vi "main.vi"() -> ()   [LabVIEW 2023]
uses:
  <vilib>/vision/Image Controls.llb/IMAQ Image.ctl
  <vilib>/vision/NI_Vision_Development_Module.lvlib
  <vilib>/vision/Pattern Matching.llb/IMAQ Match Range Setting.ctl
  <vilib>/vision/Shape Detection.llb/ShapeDetectionMatchOptions.ctl
  <vilib>/addons/database/NI_Database_API.lvlib
  <vilib>/addons/database/Command.llb/Cmd Set Parameter Value (C).vi
  <vilib>/addons/database/Connection.llb/DB Tools Open Connec (String).vi
  <vilib>/addons/database/Command.llb/Cmd Execute.vi
  <vilib>/addons/database/Recordset.llb/Rec Destroy - Command.vi
  <vilib>/addons/database/Command.llb/Cmd Delete.vi
panel:
  in  "Parameterized SQL query":string="insert into inserttable (querytype, device, numsamples) values ('parameterized sql query', ?, ?) "
  in  "Analiza Pythongowa":bool
  out "Shape Report":T1(array[cluster]) {"Score" format="%.2f"; "Centroid"."y" format="%.2f"; "Centroid"."x" format="%.2f"}
  out "Triangles":i32
  out "String":string
  out "Rectangles":i32
  out "Circles":i32
  out "Obraz":T2(plugin-control)
  in  "Output Path":path
  in  "Input Path":path=path "C:/Users/kacpe/Desktop/OSP/testp.png"
  in  "Refresh Button":bool
  in  "Process Stop Button":bool
  in  "Save As Button":bool
  in  "Analiza Labview":bool
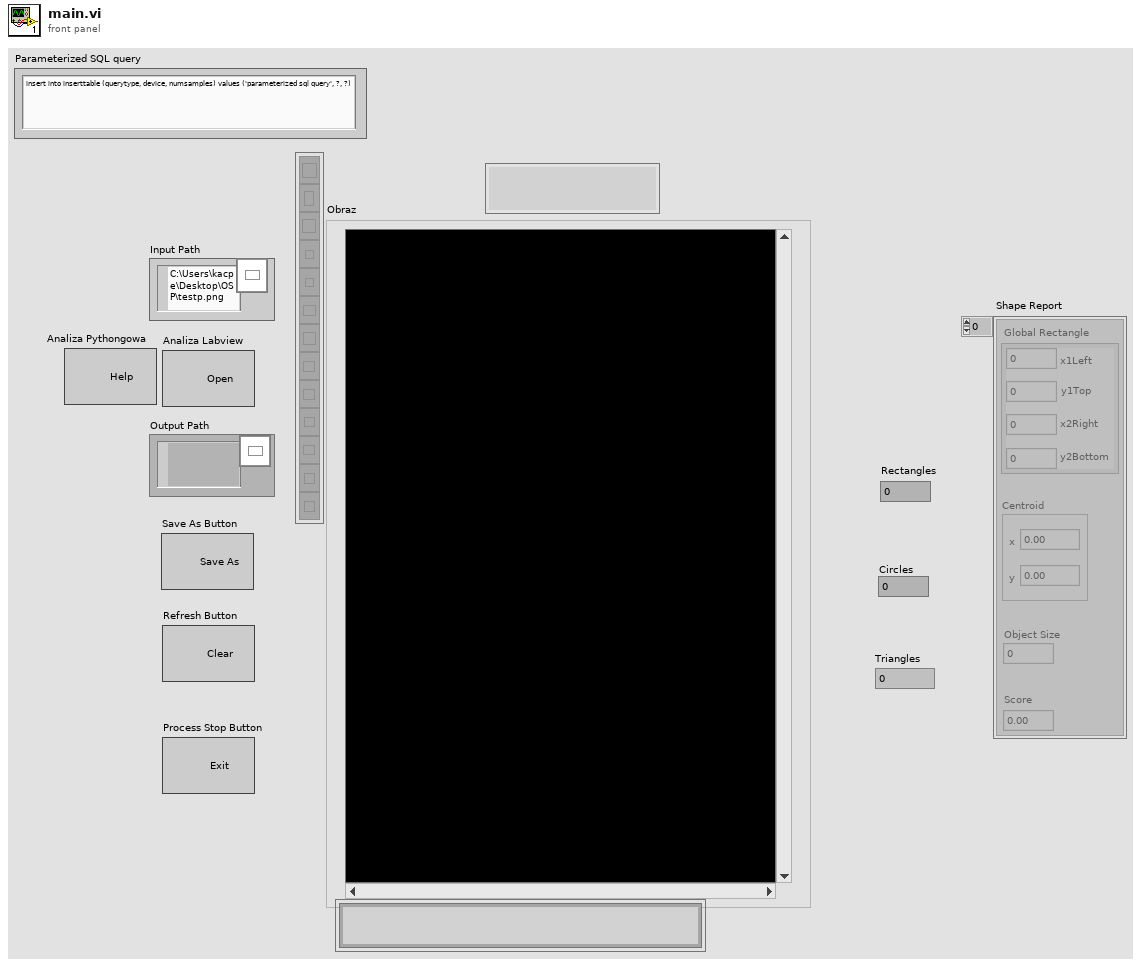
[diagram p1: front panel]
types:
  T1 = cluster{"Global Rectangle":cluster{"x1Left":i32, "y1Top":i32, "x2Right":i32, "y2Bottom":i32}, "Centroid":cluster{"x":sgl, "y":sgl}, "Object Size":u32, "Score":dbl}[]
  T2 = typedef "IMAQ Image.ctl" = refnum<image>
  T3 = enum32{"Invalid", "Standard", "Closed", "Hidden", "Minimized", "Maximized"}
  T4 = enum32{"invalid app kind", "Development System", "Run Time System", "Student Edition", "Embedded LabVIEW", "Evaluation", "Custom"}
  T5 = cluster{"Left":i32, "Top":i32, "Right":i32, "Bottom":i32}
  T6 = cluster{"Position":cluster{"x":sgl, "y":sgl}, "Angle":sgl, "Scale":sgl, "Score":sgl, "Bounding Box":cluster{"x":sgl, "y":sgl}[]}[]
  T7 = cluster{"Position":cluster{"X":sgl, "Y":sgl}, "Radius":dbl, "Score":dbl}[]
  T8 = cluster{"Min Width":dbl, "Max Width":dbl, "Min Height":dbl, "Max Height":dbl}
  T9 = cluster{"Core":cluster{"Current VI Reference":refnum<vi>, "Close Panel on Exit?":bool}, "Obraz":T2, enum16{"null", "kwadrat", "kolo", "trojkat"}, "Rectangles":cluster{"Corners":cluster{"X":sgl, "Y":sgl}[], "Angle":dbl, "Width":dbl, "Height":dbl, "Score":dbl}[], "Circles":cluster{"Position":cluster{"X":sgl, "Y":sgl}, "Radius":dbl, "Score":dbl}[], "Matches (pixel)":cluster{"Position":cluster{"x":sgl, "y":sgl}, "Angle":sgl, "Scale":sgl, "Score":sgl, "Bounding Box":cluster{"x":sgl, "y":sgl}[]}[], "Znak":string, "Input Path":path, "Python cords":cluster{"Left":i32, "Top":i32, "Right":i32, "Bottom":i32}}
  T10 = cluster{"Corners":cluster{"X":sgl, "Y":sgl}[], "Angle":dbl, "Width":dbl, "Height":dbl, "Score":dbl}[]
  T11 = cluster{"Current VI Reference":refnum<vi>, "Close Panel on Exit?":bool}
  T12 = cluster{"Position":cluster{"x":sgl, "y":sgl}, "Angle":sgl, "Scale":sgl, "Score":sgl, "Bounding Box":cluster{"x":sgl, "y":sgl}[]}
  T13 = typedef "ShapeDetectionMatchOptions.ctl" = cluster{"Rotation":bool, "Scale":bool, "Occlusion":bool, "Range Settings":T14[]}
  T14 = typedef "IMAQ Match Range Setting.ctl" = cluster{"Match Constraints":u32, "Min":dbl, "Max":dbl}
  T15 = typedef "Image Type" = u32
  T16 = typedef "NI_Database_API.lvlib/Conn ObjectReference.ctl" = refnum<k1>
  T17 = typedef "NI_Database_API.lvlib/Cmd ObjectReference.ctl" = refnum<k1>
  T18 = typedef "NI_Database_API.lvlib/Cmd-Rec Object Reference.ctl" = refnum<k1>
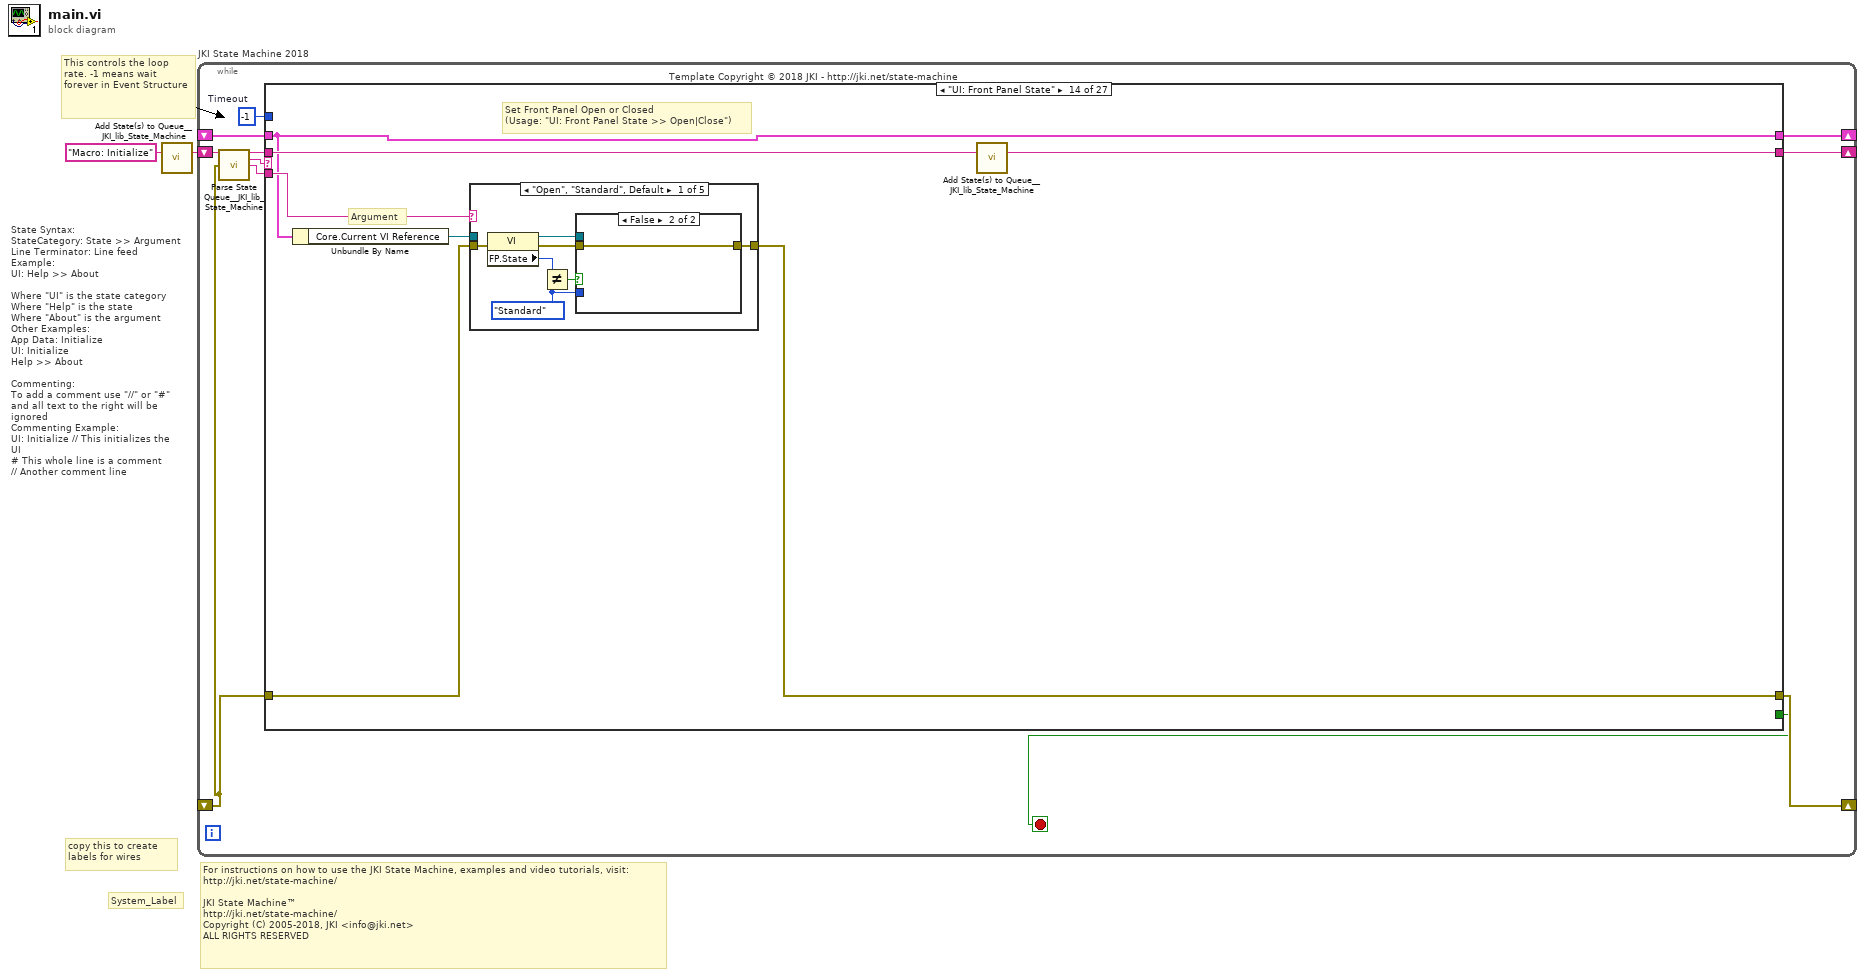
[diagram p0: block diagram]
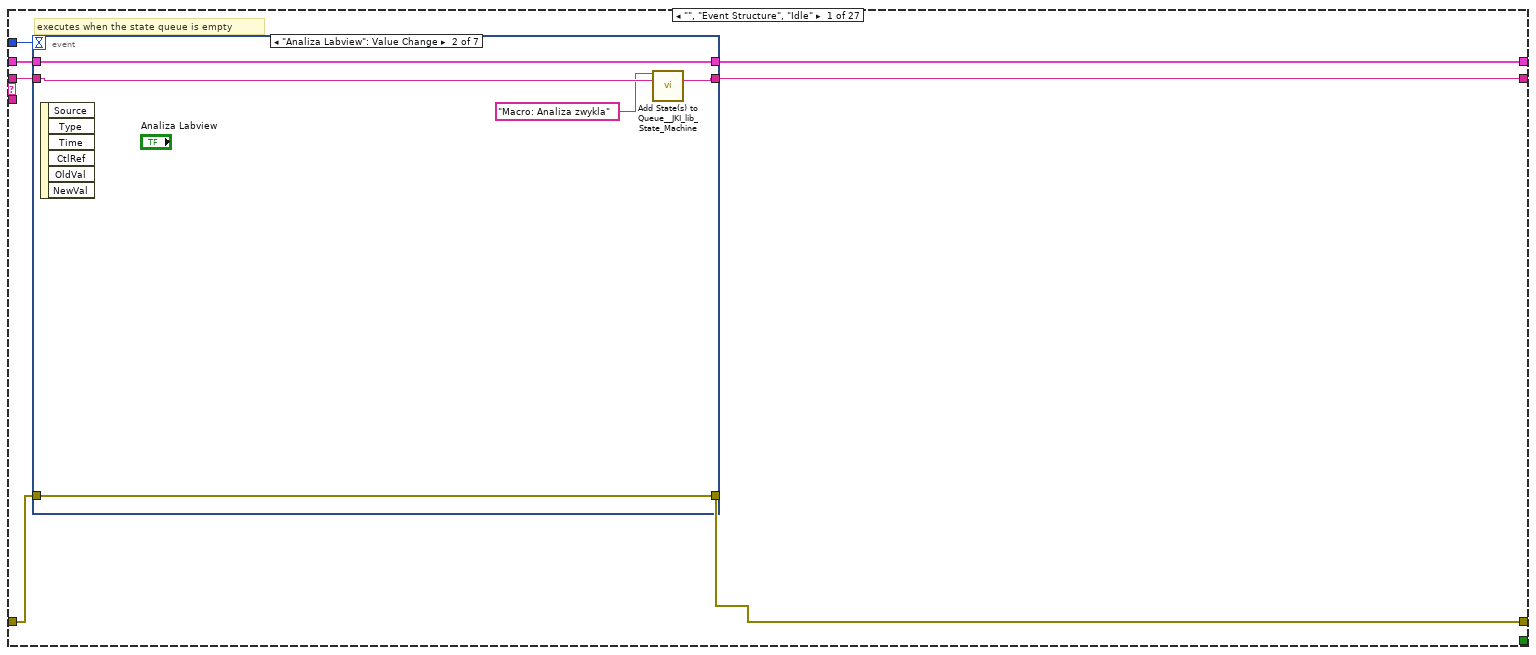
[diagram p2: hidden frame]
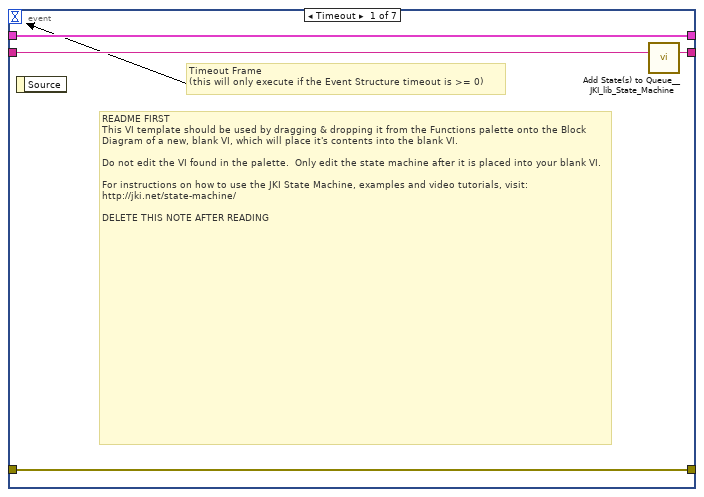
[diagram p3: hidden frame]
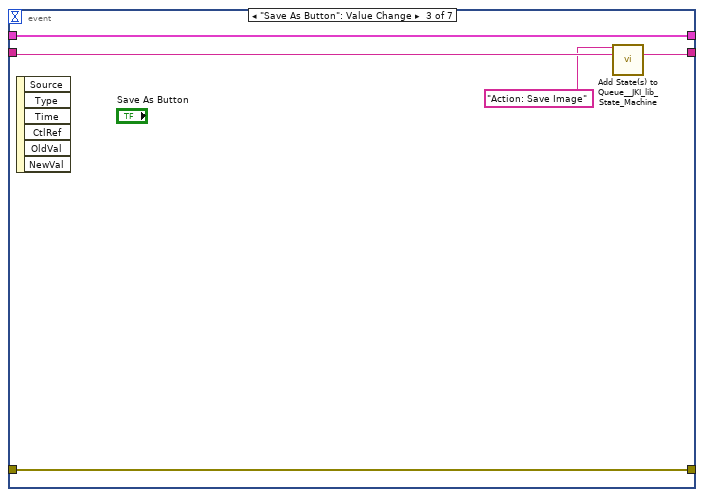
[diagram p4: hidden frame]
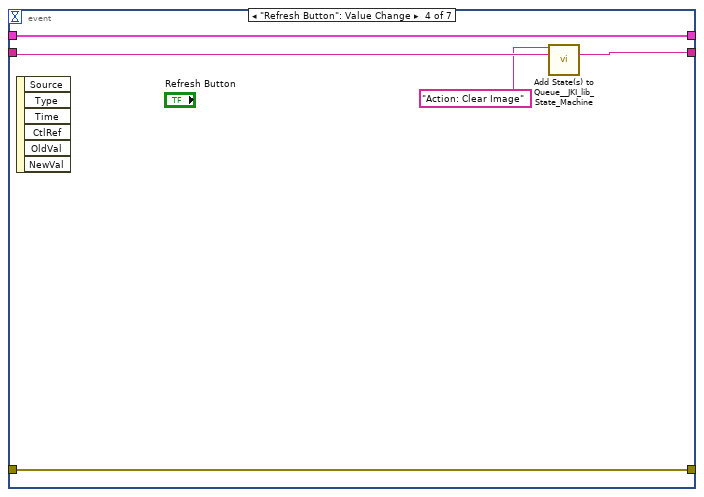
[diagram p5: hidden frame]
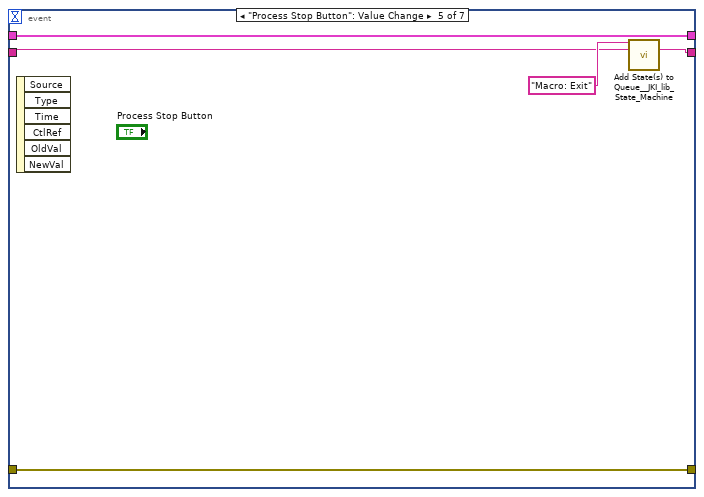
[diagram p6: hidden frame]
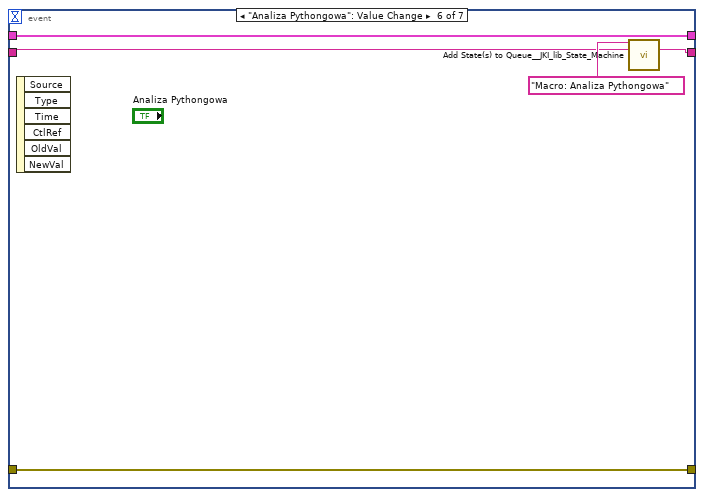
[diagram p7: hidden frame]
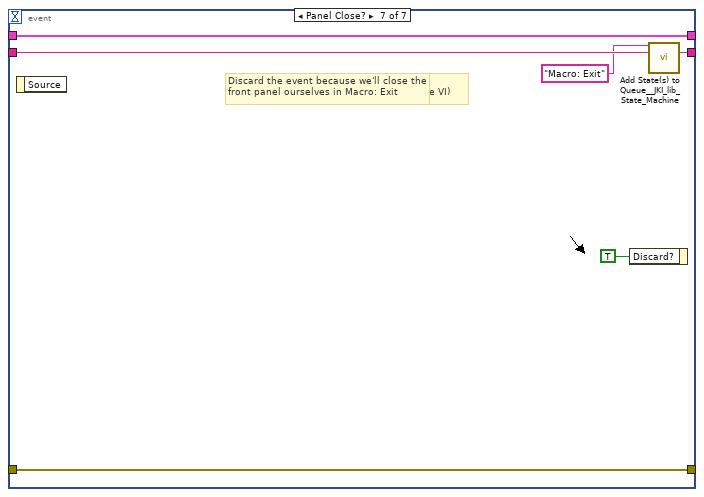
[diagram p8: hidden frame]
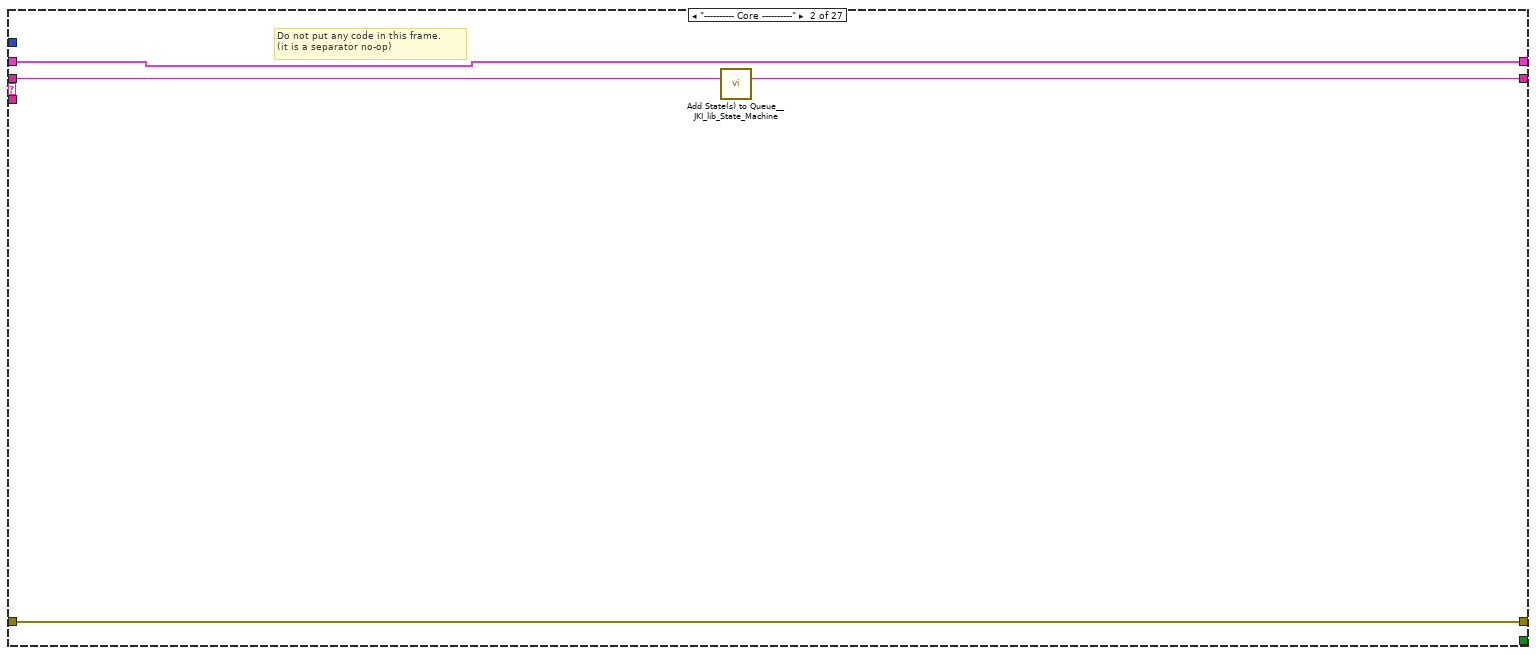
[diagram p9: hidden frame]
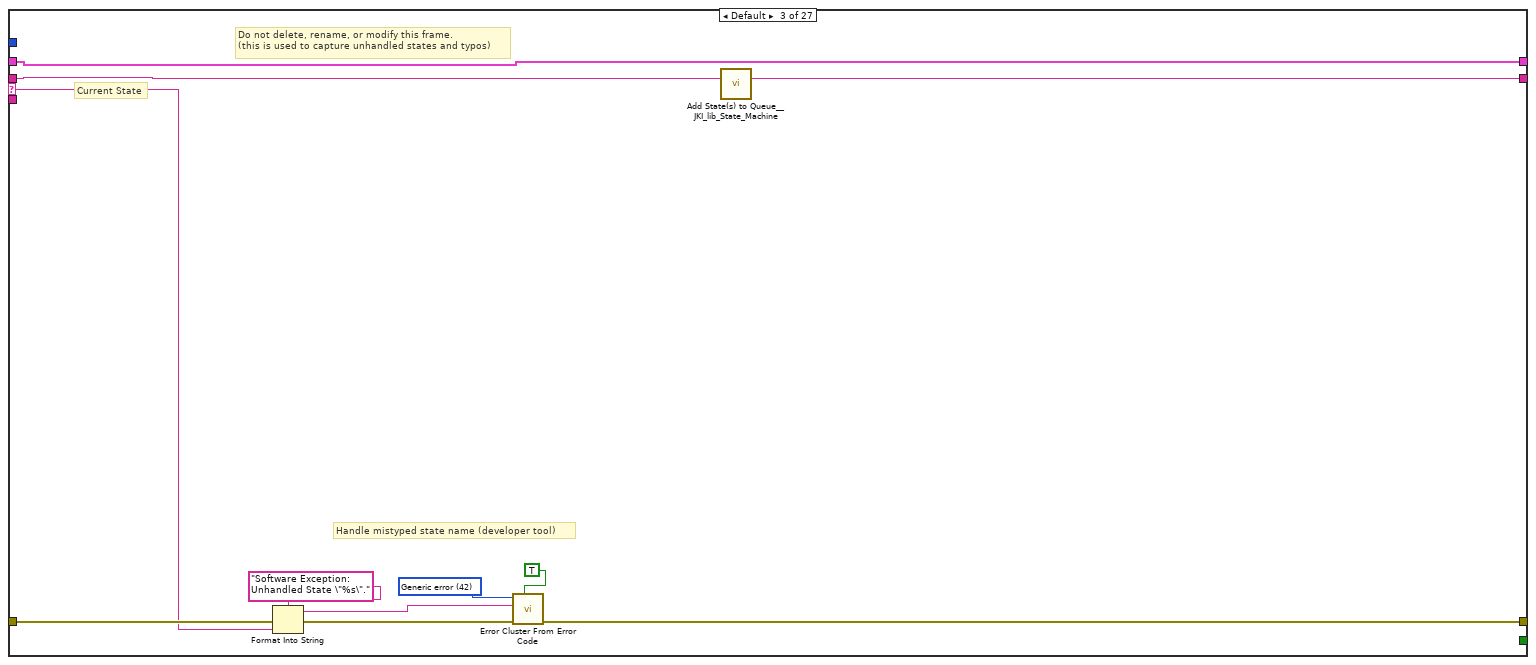
[diagram p10: hidden frame]
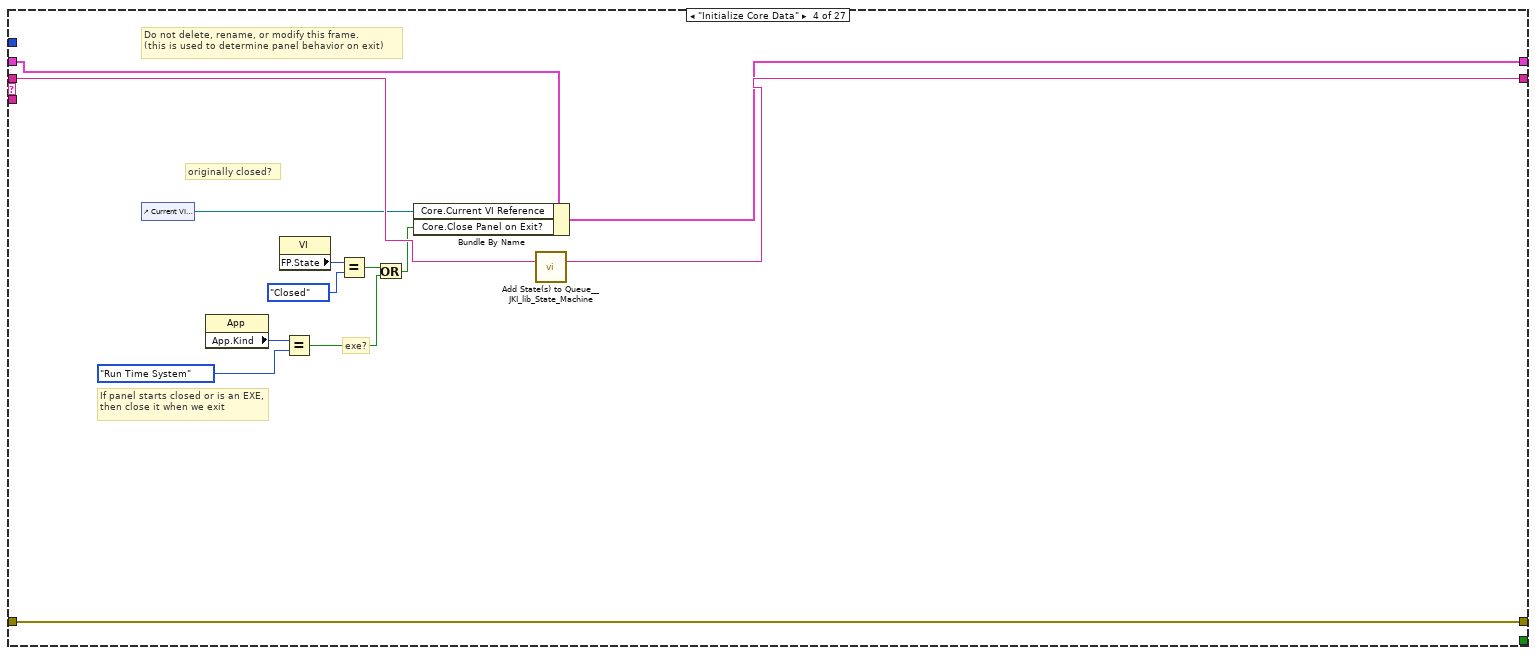
[diagram p11: hidden frame]
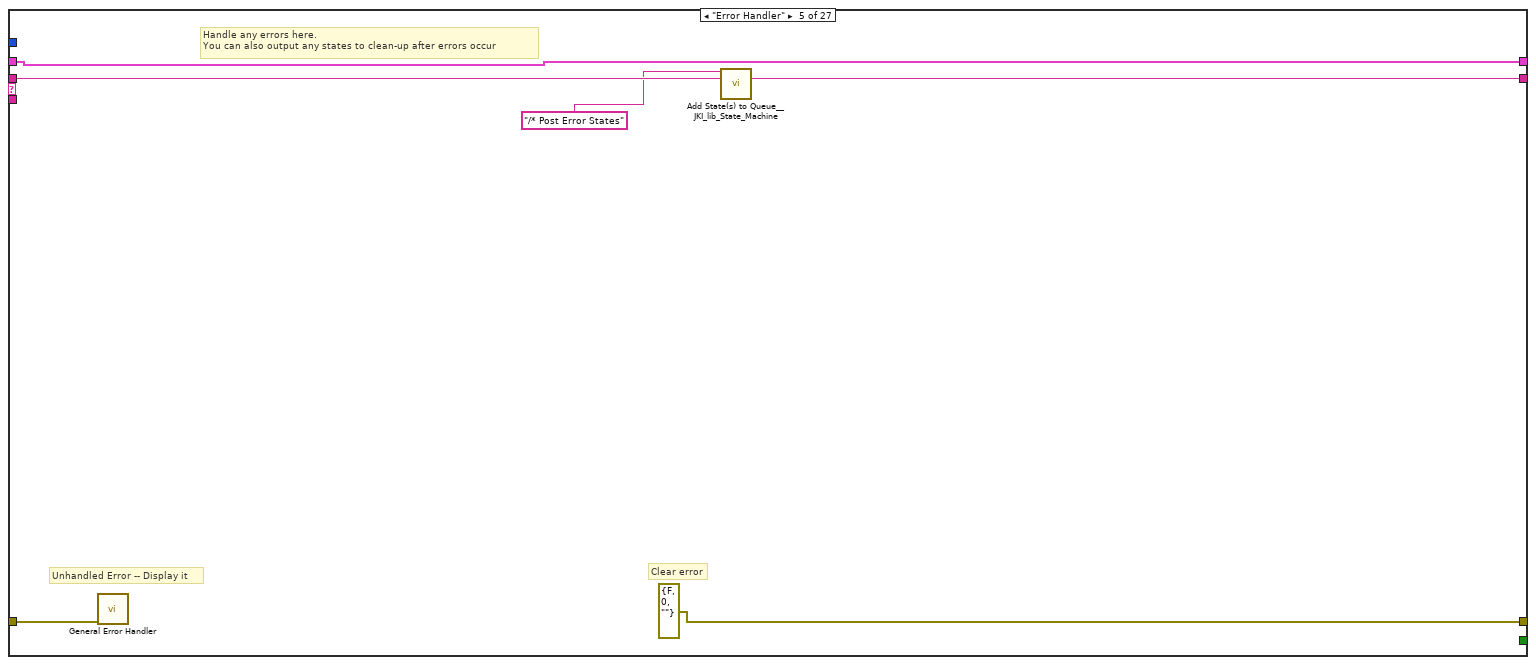
[diagram p12: hidden frame]
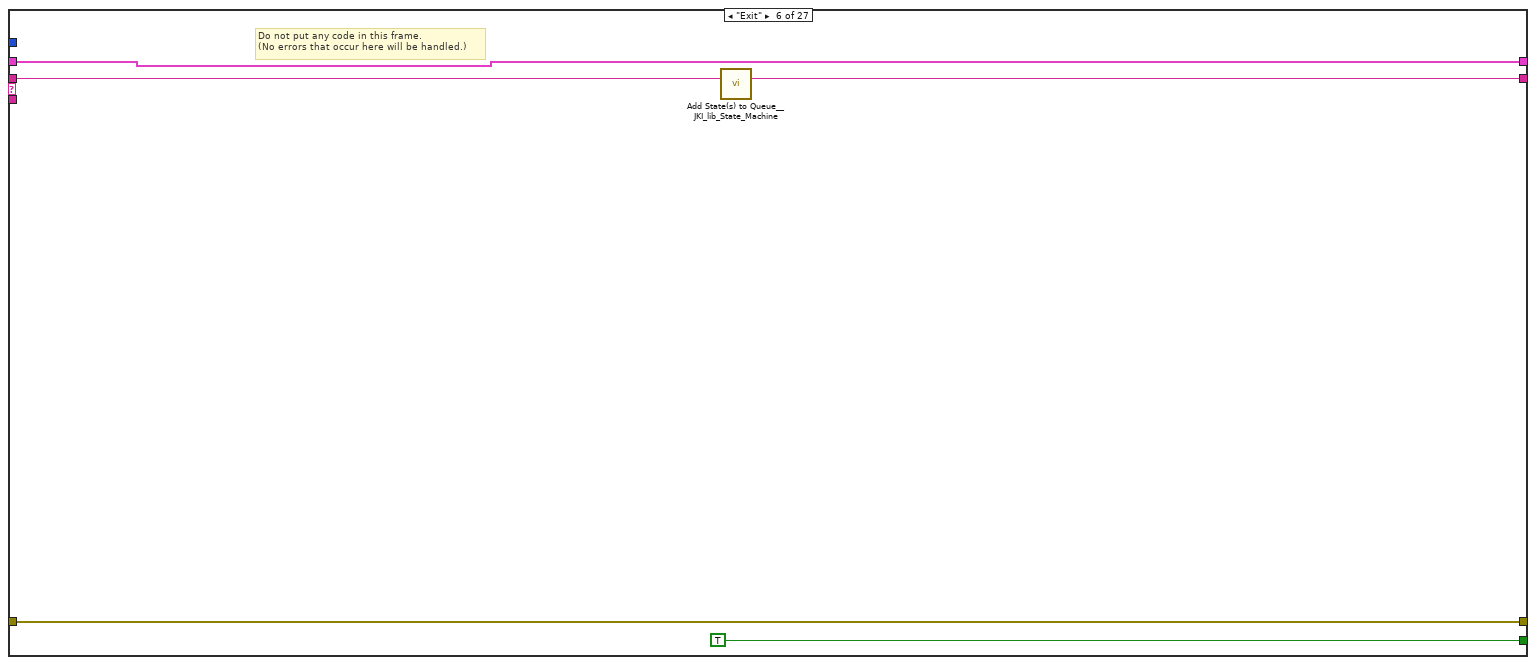
[diagram p13: hidden frame]
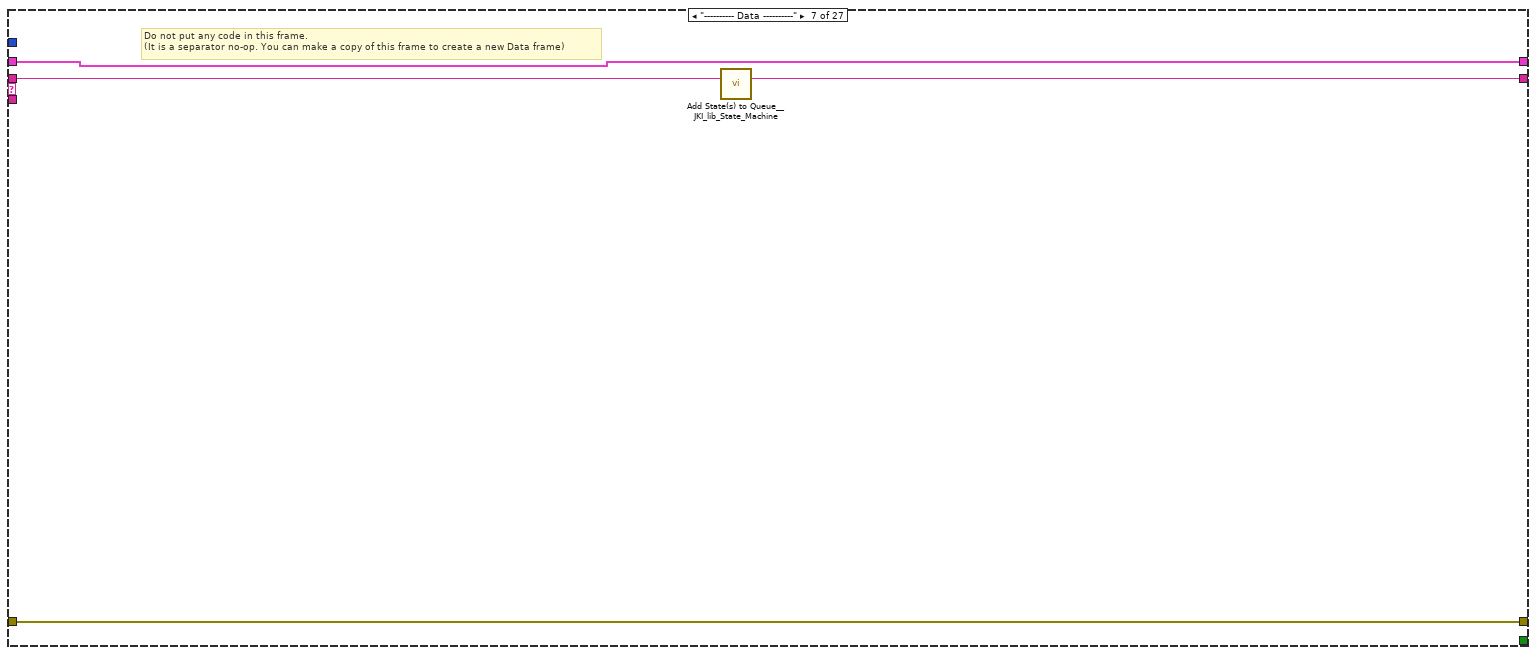
[diagram p14: hidden frame]
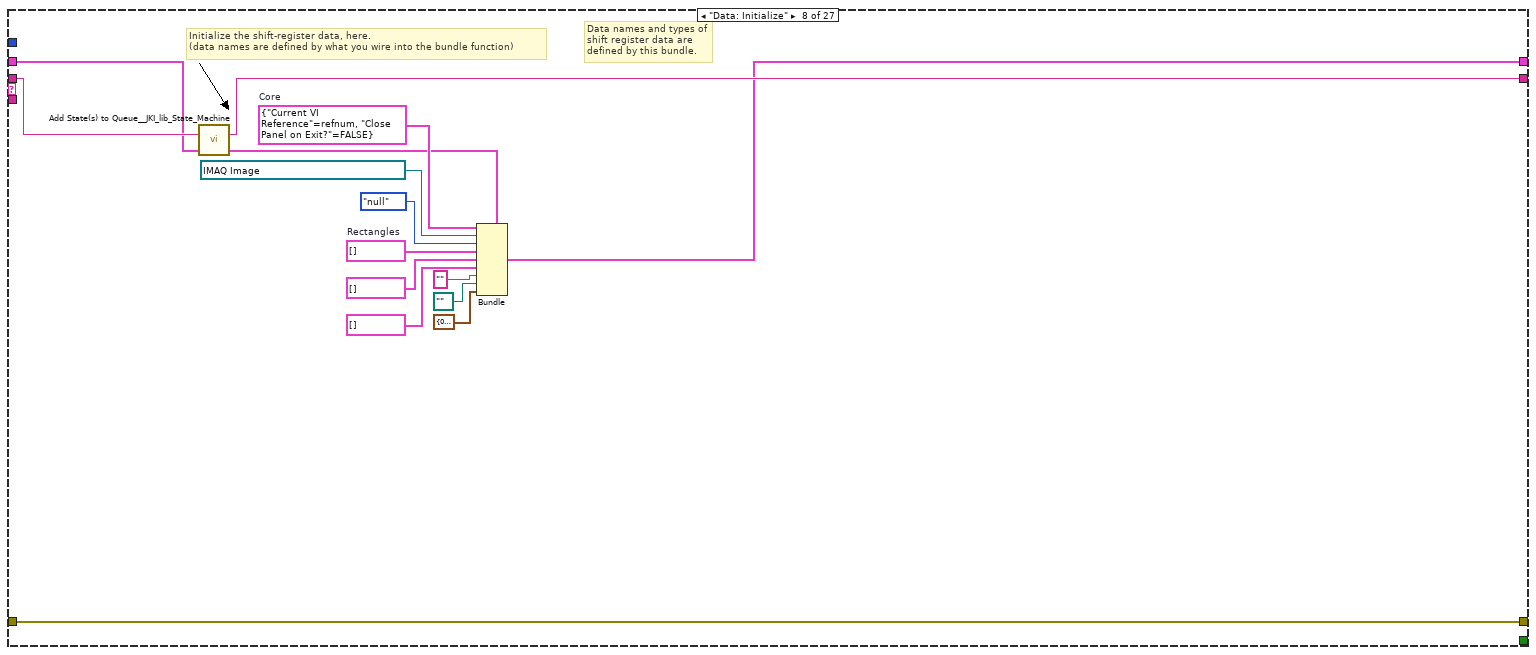
[diagram p15: hidden frame]
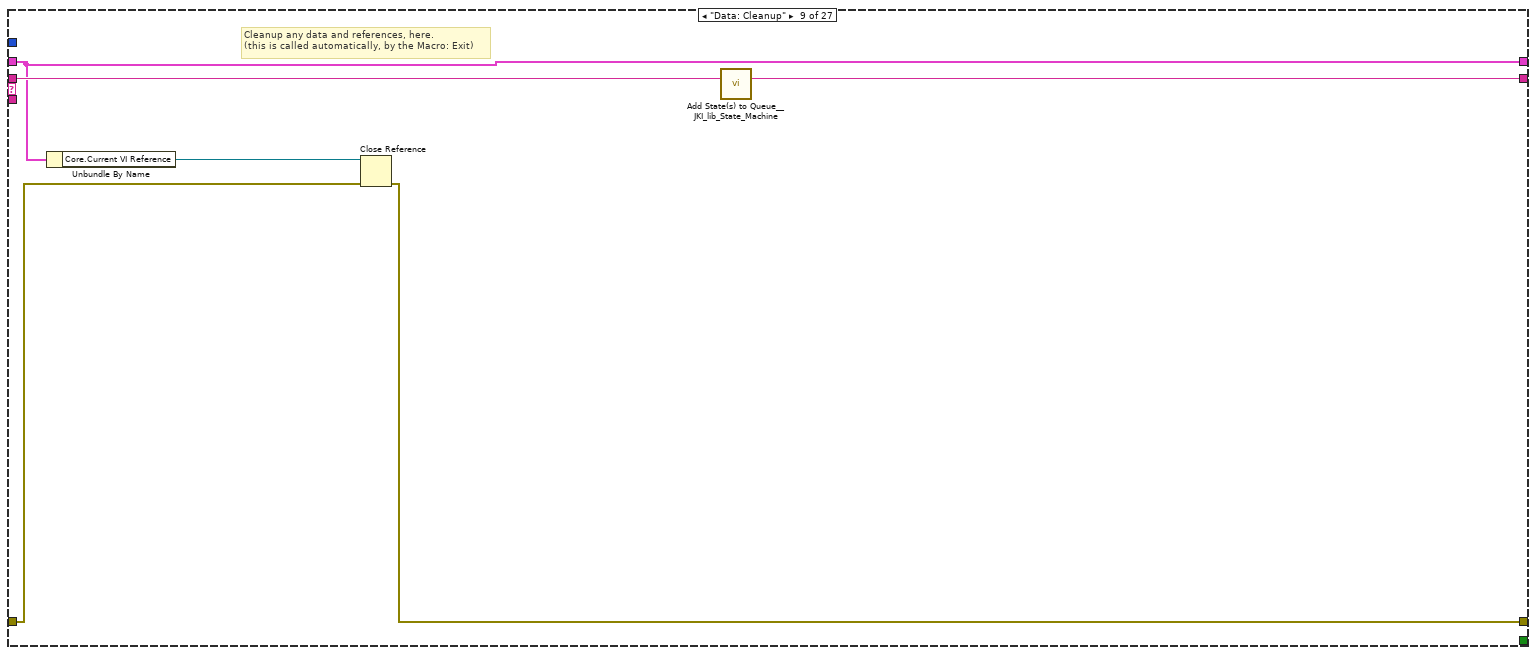
[diagram p16: hidden frame]
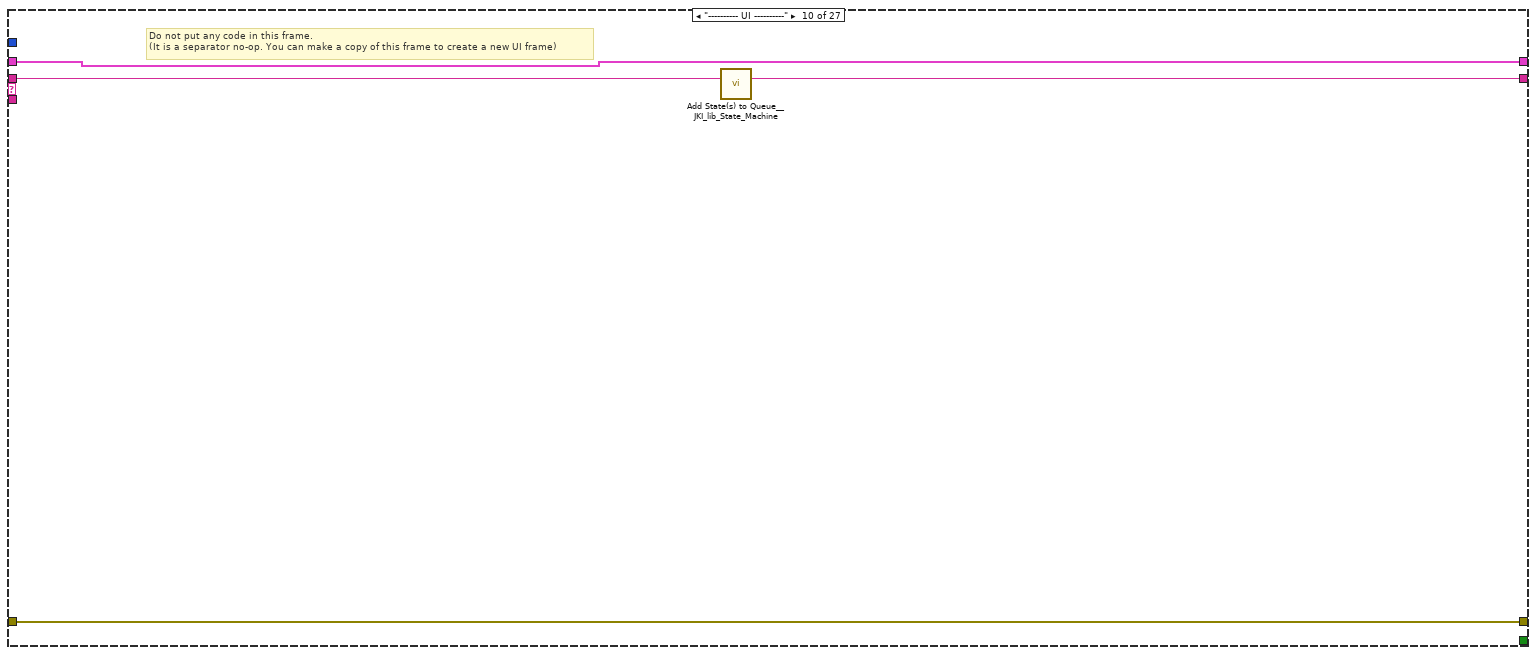
[diagram p17: hidden frame]
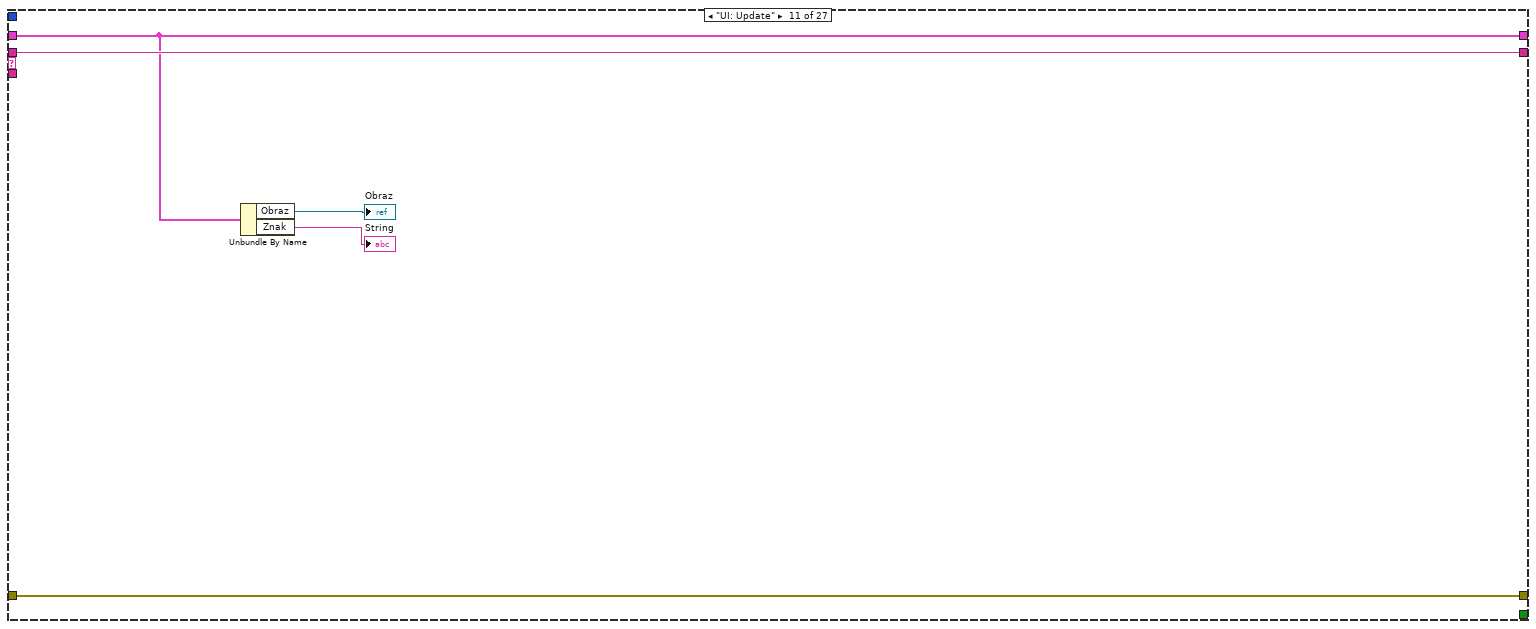
[diagram p18: hidden frame]
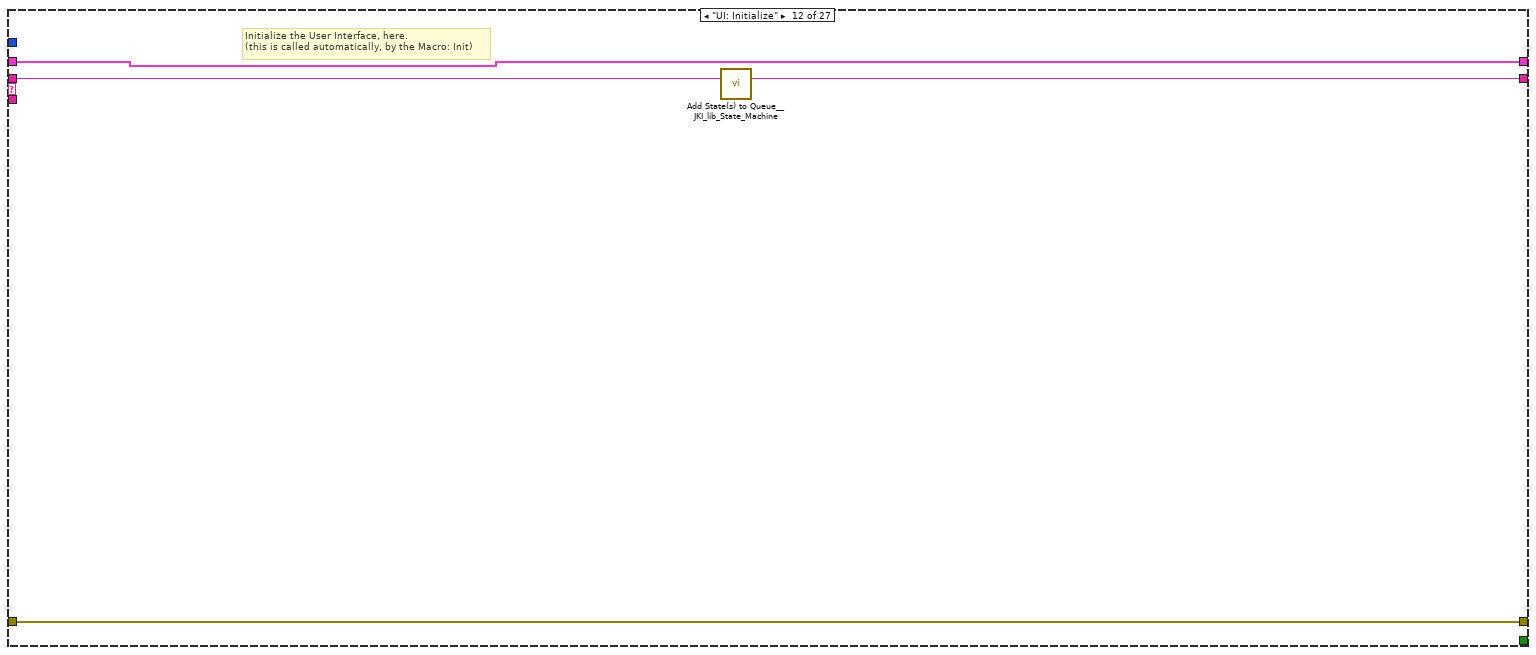
[diagram p19: hidden frame]
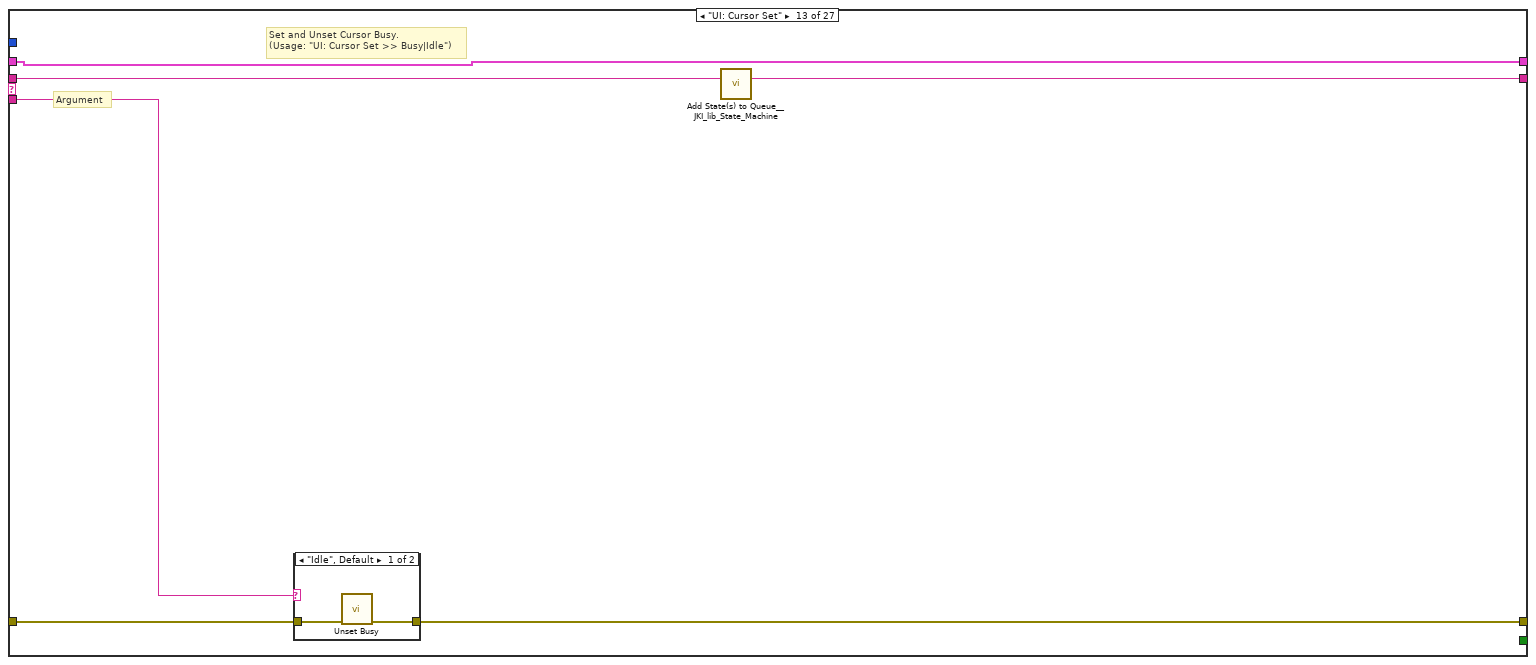
[diagram p20: hidden frame]
diagram:
  # "For instructions on how to use the JKI State Machine, examples and video tutorials, visit:\nhttp://jki.net/state-machine/\n\nJKI State Machine™\nhttp://jki.net/state-machine/\nCopyright (C) 2005-2018, JKI <info@jki.net>\nALL RIGHTS RESERVED"
  # "State Syntax:\nStateCategory: State >> Argument\nLine Terminator: Line feed\nExample:\nUI: Help >> About\n\nWhere \"UI\" is the state category\nWhere \"Help\" is the state\nWhere \"About\" is the argument\nOther Examples:\nApp Data: Initialize\nUI: Initialize\nHelp >> About\n\nCommenting:\nTo add a comment use \"//\" or \"#\" and all text to the right will be ignored\nCommenting Example:\nUI: Initialize // This initializes the UI\n# This whole line is a comment\n// Another comment line"
  # "copy this to create labels for wires"
  # "This controls the loop rate. -1 means wait forever in Event Structure"
  # "System_Label"
  n1 = call <vilib>:"Add State(s) to Queue__JKI_lib_State_Machine.vi"("State(s) in (\"\")"="Macro: Initialize") -> ("States Out"=w2:string)  [unwired: 14 in]
  n2 = while "JKI State Machine 2018" {
    shift-right: [w6] -> _
    shift-left: _ -> [w5]
    shift-right: [w9] -> _
    shift-left: _ -> [w3]
    shift-right: [w8] -> _
    shift-left: w2 -> [w10]
    stop <- w7 stop-if-true
    w4 = -1  # Timeout
    # "Template Copyright © 2018 JKI - http://jki.net/state-machine"
    n3 = call <vilib>:"Parse State Queue__JKI_lib_State_Machine.vi"("State Queue"=w10, "Error In (no error)"=w3) -> ("Remaining States"=w12:string, "Current State"=w13:string, "Arguments"=w11:string)  [unwired: 11 in]
    n4 = case shown="\"UI: Front Panel State\"" w13 {
      selector: w13 -> [_ _ w60 _ _ _ _ _ _ _ _ _ _ _ _ _ _ _ _ _ _ _ _ _ _ _ _]
      tunnel: w12 -> [w20 w59 w64 w83 w89 w94 w98 w112 w118 w122 w126 w131 w137 w148 w212 w217 w222 w227 w237 w241 w276 w291 w353 w363 w370 w397 w405]
      tunnel: w11 -> [_ _ _ _ _ _ _ _ _ _ _ _ w132 w143 _ _ _ _ _ _ _ _ _ _ _ _ _]
      tunnel: w5 -> [w18 w56 w62 w72 w86 w92 w95 w100 w114 w119 w125 w129 w135 w142 w209 w214 w219 w224 w229 w238 w264 w283 w332 w355 w365 w373 w400]
      tunnel: [w17 w57 w66 w81 errorcluster {"status"=FALSE, "code"=0, "source"=""} ("error out") w91 w96 w110 w115 w120 w127 w128 w133 w145 w210 w215 w220 w225 w235 w239 w266 w288 w351 w358 w368 w375 w403] -> w9
      tunnel: w3 -> [w16 w57 w65 w81 w85 w91 w96 w110 w116 w120 w127 w128 w134 w146 w210 w215 w220 w225 w235 w239 w269 w287 w350 w358 w367 w374 w403]
      tunnel: [w19 w58 w63 w82 w88 w93 w97 w111 w117 w121 w126 w130 w136 w147 w211 w216 w221 w226 w236 w240 w276 w290 w352 w362 w369 w396 w404] -> w8
      tunnel: [_ _ _ _ _ TRUE _ _ _ _ _ _ _ _ _ _ _ _ _ _ _ _ _ _ _ _ _] -> w7
      tunnel: [w15 w56 w62 w71 w86 w92 w95 w99 w114 w119 w125 w129 w135 w142 w209 w214 w219 w224 w229 w238 w265 w284 w333 w356 w365 w373 w401] -> w6
      tunnel: w4 -> [w14 _ _ _ _ _ _ _ _ _ _ _ _ _ _ _ _ _ _ _ _ _ _ _ _ _ _]
      frame "", "Event Structure", "Idle" {
        # "executes when the state queue is empty"
        n5 = event shown="[1] \"Analiza Labview\": Value Change" {
          selector: _ -> [_ _ _ _ _ _ _]
          dyn-events: _ -> [_ _ _ _ _ _ _]
          timeout: w14 -> [_ _ _ _ _ _ _]
          tunnel: w20 -> [w24 w27 w31 w36 w41 w46 w55]
          tunnel: [w23 w28 w32 w37 w43 w48 w54] -> w19
          tunnel: w18 -> [w21 w29 w34 w39 w44 w49 w52]
          tunnel: [w22 w25 w33 w38 w40 w45 w53] -> w17
          tunnel: w16 -> [w22 w25 w33 w38 w40 w45 w53]
          tunnel: [w21 w29 w34 w39 w44 w49 w52] -> w15
          event Timeout {
            # "README FIRST\nThis VI template should be used by dragging & dropping it from the Functions palette onto the Block Diagram of a new, blank VI, which will place it's contents into the blank VI.\n\nDo not edit the VI found in the palette.  Only edit the state machine after it is placed into your blank VI.\n\nFor instructions on how to use the JKI State Machine, examples and video tutorials, visit:\nhttp://jki.net/state-machine/\n\nDELETE THIS NOTE AFTER READING"
            # "Timeout Frame\n(this will only execute if the Event Structure timeout is >= 0)"
            n6 = event-data() -> ()  [unwired: 1 in, 1 out]
            n7 = call <vilib>:"Add State(s) to Queue__JKI_lib_State_Machine.vi"("State(s) in (\"\")"=w24) -> ("States Out"=w23:string)  [unwired: 14 in]
          }
          event "Analiza Labview": Value Change {
            n8 = event-data() -> ()  [unwired: 1 in, 6 out]
            n9 = call <vilib>:"Add State(s) to Queue__JKI_lib_State_Machine.vi"("State(s) in Front (\"\")"="Macro: Analiza zwykla" ("State(s) in Front (\"\")"), "State(s) in (\"\")"=w27) -> ("States Out"=w28:string)  [unwired: 13 in]
          }
          event "Save As Button": Value Change {
            n10 = event-data() -> ()  [unwired: 1 in, 6 out]
            n11 = call <vilib>:"Add State(s) to Queue__JKI_lib_State_Machine.vi"("State(s) in Front (\"\")"="Action: Save Image" ("State(s) in Front (\"\")"), "State(s) in (\"\")"=w31) -> ("States Out"=w32:string)  [unwired: 13 in]
          }
          event "Refresh Button": Value Change {
            n12 = event-data() -> ()  [unwired: 1 in, 6 out]
            n13 = call <vilib>:"Add State(s) to Queue__JKI_lib_State_Machine.vi"("State(s) in Front (\"\")"="Action: Clear Image" ("State(s) in Front (\"\")"), "State(s) in (\"\")"=w36) -> ("States Out"=w37:string)  [unwired: 13 in]
          }
          event "Process Stop Button": Value Change {
            n14 = event-data() -> ()  [unwired: 1 in, 6 out]
            n15 = call <vilib>:"Add State(s) to Queue__JKI_lib_State_Machine.vi"("State(s) in Front (\"\")"="Macro: Exit", "State(s) in (\"\")"=w41) -> ("States Out"=w43:string)  [unwired: 13 in]
          }
          event "Analiza Pythongowa": Value Change {
            n16 = event-data() -> ()  [unwired: 1 in, 6 out]
            n17 = call <vilib>:"Add State(s) to Queue__JKI_lib_State_Machine.vi"("State(s) in Front (\"\")"="Macro: Analiza Pythongowa", "State(s) in (\"\")"=w46) -> ("States Out"=w48:string)  [unwired: 13 in]
          }
          event Panel Close? {
            # "Discard the event because we'll close the front panel ourselves in Macro: Exit"
            # "Close Panel button (pressed) Event\n(this executes Macro: Exit to terminate the VI)"
            n18 = event-data() -> ()  [unwired: 1 in, 1 out]
            n19 = event-data("Discard?"=TRUE) -> ()  [unwired: 1 in, 1 out]
            n20 = call <vilib>:"Add State(s) to Queue__JKI_lib_State_Machine.vi"("State(s) in Front (\"\")"="Macro: Exit", "State(s) in (\"\")"=w55) -> ("States Out"=w54:string)  [unwired: 13 in]
          }
        }
      }
      frame "---------- Core ----------" {
        # "Do not put any code in this frame.\n(it is a separator no-op)"
        n21 = call <vilib>:"Add State(s) to Queue__JKI_lib_State_Machine.vi"("State(s) in (\"\")"=w59) -> ("States Out"=w58:string)  [unwired: 14 in]
      }
      frame Default {
        w69 = 42 items=["No error", "Argument error", "Memory is full", "Out of zone", "End of file", "File already open", "Generic file I/O error", "File not found", "File permission error", "Disk is full", "Duplicate path", "Too many files open", "System feature not enabled", "Resource file not found", "Cannot add resource", "Resource not found", "Image not found", "Image memory error", "Pen does not exist", "Config type invalid", "Config token not found", "Config parse error", "Config memory error", "Bad external code format", "Bad external code offset", "External code not present", "Null window", "Destroy window error", "Null menu", "Print aborted", "Bad print record", "Print driver error", "Windows error during printing", "Memory error during printing", "Print dialog error", "Generic print error", "Invalid device refnum", "Device not found", "Device parameter error", "Device unit error", "Cannot open device", "Device call aborted", "Generic error", "Cancelled by user", "Object ID too low", "Object ID too high", "Object not in heap", "Unknown heap", "Unknown object (invalid DefProc)", "Unknown object (DefProc not in table)", "Message out of range", "Invalid (null) method", "Unknown message", "Manager call not supported", "Bad address", "Network operation in progress", "Network operation timed out", "Connection is busy", "Network attribute not supported", "Network error", "Address in use", "System out of memory", "Connection aborted", "Connection refused", "Not connected", "Already connected", "Connection closed", "Initialization error (interapplication manager)", "Bad occurrence", "Wait on unbound occurrence handler", "Occurrence queue overflow", "Datalog type conflict", "Unused", "Unrecognized type (interapplication manager)", "Memory corrupt", "Failed to make temporary DLL", "Old CIN version", "Drag socket not found", "Failed to load drop-object", "Failed to register OLE object", "Failed to release OLE object", "Format specifier type mismatch", "Unknown format specifier", "Too few format specifiers", "Too many format specifiers", "Scan failed", "Newer CIN version", "Error converting to variant", "Runtime menu error", "Password tampered", "Variant attribute not found", "Incompatible variant data type", "Event data is not available", "Event Store is not present", "Occurrence is not found", "Event Queue is not created", "Event info is not available", "Refnum passed is NULL", "Error retrieving Class GUID", "Error retrieving CoClass GUID", "Error retrieving TypeLib GUID.", "Bad built application magic bytes.", "Specific driver is different from the specific driver associated with the Logical Name.", "There is no session opened to the class driver.", "Max Error", "MAX - Error with config objects", "MAX - Error loading configuration", "MAX - Group not supported"]
        # "Current State"
        # "Do not delete, rename, or modify this frame.\n(this is used to capture unhandled states and typos)"
        # "Handle mistyped state name (developer tool)"
        n22 = Format Into String(format string="Software Exception: Unhandled State \"%s\"." ("message"), error in=w65, w60) -> (resulting string=w68:string, error out=w67:errorcluster)  [unwired: 1 in]
        n23 = call <vilib>:"Error Cluster From Error Code.vi"("show call chain? (False)"=TRUE, "error in (no error)"=w67, "error message (\"\")"=w68, "error code (0)"=w69) -> ("error out"=w66:errorcluster)  [unwired: 5 in]
        n24 = call <vilib>:"Add State(s) to Queue__JKI_lib_State_Machine.vi"("State(s) in (\"\")"=w64) -> ("States Out"=w63:string)  [unwired: 14 in]
      }
      frame "Initialize Core Data" {
        # "Do not delete, rename, or modify this frame.\n(this is used to determine panel behavior on exit)"
        # "originally closed?"
        # "exe?"
        # "If panel starts closed or is an EXE, then close it when we exit"
        n25 = control-ref of="Current VI Reference"() -> (w76:refnum<vi>)
        n26 = property class="App"() -> ("App.Kind"=w80:T4)  [unwired: 2 in, 2 out]
        n27 = property class="VI"() -> ("FP.State"=w75:T3)  [unwired: 2 in, 2 out]
        n28 = Equal?(x=w80, y=T4."Run Time System" ("Application:Kind")) -> (x = y?=w78:bool)
        n29 = Equal?(x=w75, y=T3."Closed" ("Front Panel Window:State")) -> (x = y?=w73:bool)
        n30 = Or(x=w73, y=w78) -> (x .or. y?=w77:bool)
        n31 = Bundle By Name(cluster=w72, "Core.Current VI Reference"=w76, "Core.Close Panel on Exit?"=w77) -> (w71:T9)
        n32 = call <vilib>:"Add State(s) to Queue__JKI_lib_State_Machine.vi"("State(s) in (\"\")"=w83) -> ("States Out"=w82:string)  [unwired: 14 in]
      }
      frame "Error Handler" {
        # "Unhandled Error -- Display it"
        # "Handle any errors here.\nYou can also output any states to clean-up after errors occur"
        # "Clear error"
        n33 = call <vilib>:"General Error Handler.vi"("error in (no error)"=w85) -> ()  [unwired: 10 in, 5 out]
        n34 = call <vilib>:"Add State(s) to Queue__JKI_lib_State_Machine.vi"("State(s) in Front (\"\")"="/* Post Error States", "State(s) in (\"\")"=w89) -> ("States Out"=w88:string)  [unwired: 13 in]
      }
      frame "Exit" {
        # "Do not put any code in this frame.\n(No errors that occur here will be handled.)"
        n35 = call <vilib>:"Add State(s) to Queue__JKI_lib_State_Machine.vi"("State(s) in (\"\")"=w94) -> ("States Out"=w93:string)  [unwired: 14 in]
      }
      frame "---------- Data ----------" {
        # "Do not put any code in this frame.\n(It is a separator no-op. You can make a copy of this frame to create a new Data frame)"
        n36 = call <vilib>:"Add State(s) to Queue__JKI_lib_State_Machine.vi"("State(s) in (\"\")"=w98) -> ("States Out"=w97:string)  [unwired: 14 in]
      }
      frame "Data: Initialize" {
        w106 = T10 []  # Rectangles
        w109 = T11 {"Current VI Reference"=refnum, "Close Panel on Exit?"=FALSE}  # Core
        # "Data names and types of shift register data are defined by this bundle."
        # "Initialize the shift-register data, here.\n(data names are defined by what you wire into the bundle function)"
        n37 = call <vilib>:"Add State(s) to Queue__JKI_lib_State_Machine.vi"("State(s) in (\"\")"=w112) -> ("States Out"=w111:string)  [unwired: 14 in]
        n38 = Bundle(cluster=w100, "Core"=w109, "Obraz"=T2 refnum, enum16{"null", "kwadrat", "kolo", "trojkat"}."null", "Rectangles"=w106, "Circles"=T7 [], "Matches (pixel)"=T6 [], "Znak"="", "Input Path"=path "", "Python cords"=T5 {"Left"=0, "Top"=0, "Right"=0, "Bottom"=0}) -> (w99:T9)
      }
      frame "Data: Cleanup" {
        # "Cleanup any data and references, here.\n(this is called automatically, by the Macro: Exit)"
        n39 = Unbundle By Name(w114) -> ("Core.Current VI Reference"=w113:refnum<vi>)
        n40 = Close Reference(reference=w113, error in (no error)=w116) -> (error out=w115:errorcluster)
        n41 = call <vilib>:"Add State(s) to Queue__JKI_lib_State_Machine.vi"("State(s) in (\"\")"=w118) -> ("States Out"=w117:string)  [unwired: 14 in]
      }
      frame "---------- UI ----------" {
        # "Do not put any code in this frame.\n(It is a separator no-op. You can make a copy of this frame to create a new UI frame)"
        n42 = call <vilib>:"Add State(s) to Queue__JKI_lib_State_Machine.vi"("State(s) in (\"\")"=w122) -> ("States Out"=w121:string)  [unwired: 14 in]
      }
      frame "UI: Update" {
        n43 = Unbundle By Name(w125) -> ("Obraz"=→"Obraz":T2, "Znak"=→"String":string)
      }
      frame "UI: Initialize" {
        # "Initialize the User Interface, here.\n(this is called automatically, by the Macro: Init)"
        n44 = call <vilib>:"Add State(s) to Queue__JKI_lib_State_Machine.vi"("State(s) in (\"\")"=w131) -> ("States Out"=w130:string)  [unwired: 14 in]
      }
      frame "UI: Cursor Set" {
        # "Argument"
        # "Set and Unset Cursor Busy.\n(Usage: \"UI: Cursor Set >> Busy|Idle\")"
        n45 = case shown="\"Idle\", Default" w132 {
          tunnel: w134 -> [w139 w141]
          tunnel: [w138 w140] -> w133
          frame "Idle", Default {
            n46 = call <vilib>:"Unset Busy.vi"("error in (no error)"=w139) -> ("error out"=w138:errorcluster)  [unwired: 10 in]
          }
          frame "Busy" {
            n47 = call <vilib>:"Set Busy.vi"("error in (no error)"=w141) -> ("error out"=w140:errorcluster)  [unwired: 9 in, 1 out]
          }
        }
        n48 = call <vilib>:"Add State(s) to Queue__JKI_lib_State_Machine.vi"("State(s) in (\"\")"=w137) -> ("States Out"=w136:string)  [unwired: 14 in]
      }
      frame "UI: Front Panel State" {
        # "Argument"
        # "Set Front Panel Open or Closed\n(Usage: \"UI: Front Panel State >> Open|Close\")"
        n49 = Unbundle By Name(w142) -> ("Core.Current VI Reference"=w144:refnum<vi>)
        n50 = case shown="\"Open\", \"Standard\", Default" w143 {
          tunnel: w146 -> [w154 w167 w178 w190 w202]
          tunnel: [w155 w168 w179 w191 w203] -> w145
          tunnel: w144 -> [_ _ _ _ _]
          frame "Open", "Standard", Default {
            w149 = T3."Standard" ("State")
            n51 = property class="VI"(error in=w154) -> (reference out=w152:refnum<vi>, error out=w153:errorcluster, "FP.State"=w151:T3)  [unwired: 1 in]
            n52 = Not Equal?(x=w151, y=w149) -> (x != y?=w150:bool)
            n53 = case shown="False" w150 {
              tunnel: [w159 w161] -> w155
              tunnel: w153 -> [w158 w161]
              tunnel: w152 -> [w157 _]
              tunnel: w149 -> [w156 _]
              frame True {
                n54 = invoke class="VI" method="FP.Open"(reference=w157, error in=w158, "Activate"=TRUE, "State"=w156) -> (error out=w159:errorcluster)  [unwired: 1 in, 4 out]
              }
              frame False {
              }
            }
          }
          frame "Close", "Closed" {
            n55 = property class="VI"(error in=w167) -> (reference out=w165:refnum<vi>, error out=w166:errorcluster, "FP.State"=w163:T3)  [unwired: 1 in]
            n56 = Not Equal?(x=w163, y=T3."Closed" ("Front Panel Window:State")) -> (x != y?=w162:bool)
            n57 = case shown="True" w162 {
              tunnel: [w169 w172] -> w168
              tunnel: w166 -> [w169 w171]
              tunnel: w165 -> [_ w170]
              frame False {
              }
              frame True {
                n58 = invoke class="VI" method="FP.Close"(reference=w170, error in=w171) -> (error out=w172:errorcluster)  [unwired: 1 in, 2 out]
              }
            }
          }
          frame "Hidden", "Hide" {
            w173 = T3."Hidden" ("State")
            n59 = property class="VI"(error in=w178) -> (reference out=w176:refnum<vi>, error out=w177:errorcluster, "FP.State"=w175:T3)  [unwired: 1 in]
            n60 = Not Equal?(x=w175, y=w173) -> (x != y?=w174:bool)
            n61 = case shown="True" w174 {
              tunnel: [w183 w184] -> w179
              tunnel: w177 -> [w182 w184]
              tunnel: w176 -> [w181 _]
              tunnel: w173 -> [w180 _]
              frame True {
                n62 = invoke class="VI" method="FP.Open"(reference=w181, error in=w182, "State"=w180) -> (error out=w183:errorcluster)  [unwired: 2 in, 4 out]
              }
              frame False {
              }
            }
          }
          frame "Minimize", "Minimized" {
            w185 = T3."Minimized" ("State")
            n63 = property class="VI"(error in=w190) -> (reference out=w188:refnum<vi>, error out=w189:errorcluster, "FP.State"=w187:T3)  [unwired: 1 in]
            n64 = Not Equal?(x=w187, y=w185) -> (x != y?=w186:bool)
            n65 = case shown="True" w186 {
              tunnel: [w195 w196] -> w191
              tunnel: w189 -> [w194 w196]
              tunnel: w188 -> [w193 _]
              tunnel: w185 -> [w192 _]
              frame True {
                n66 = invoke class="VI" method="FP.Open"(reference=w193, error in=w194, "State"=w192) -> (error out=w195:errorcluster)  [unwired: 2 in, 4 out]
              }
              frame False {
              }
            }
          }
          frame "Maximize", "Maximized" {
            w197 = T3."Maximized" ("State")
            n67 = property class="VI"(error in=w202) -> (reference out=w200:refnum<vi>, error out=w201:errorcluster, "FP.State"=w199:T3)  [unwired: 1 in]
            n68 = Not Equal?(x=w199, y=w197) -> (x != y?=w198:bool)
            n69 = case shown="True" w198 {
              tunnel: [w207 w208] -> w203
              tunnel: w201 -> [w206 w208]
              tunnel: w200 -> [w205 _]
              tunnel: w197 -> [w204 _]
              frame True {
                n70 = invoke class="VI" method="FP.Open"(reference=w205, error in=w206, "State"=w204) -> (error out=w207:errorcluster)  [unwired: 2 in, 4 out]
              }
              frame False {
              }
            }
          }
        }
        n71 = call <vilib>:"Add State(s) to Queue__JKI_lib_State_Machine.vi"("State(s) in (\"\")"=w148) -> ("States Out"=w147:string)  [unwired: 14 in]
      }
      frame "---------- Macro ----------" {
        # "Do not put any code in this frame.\n(It is a separator no-op. You can make a copy of this frame to create a new Macro frame)"
        n72 = call <vilib>:"Add State(s) to Queue__JKI_lib_State_Machine.vi"("State(s) in (\"\")"=w212) -> ("States Out"=w211:string)  [unwired: 14 in]
      }
      frame "Macro: Initialize" {
        w213 = "Data: Initialize\nInitialize Core Data\nUI: Initialize\nUI: Front Panel State >> Open"  # Data: Initialize Initialize Core Data UI: Initialize UI: Front Panel State >> Open
        # "Initialization Macro\n(This is called once, when the VI starts)"
        n73 = call <vilib>:"Add State(s) to Queue__JKI_lib_State_Machine.vi"("State(s) in Front (\"\")"=w213, "State(s) in (\"\")"=w217) -> ("States Out"=w216:string)  [unwired: 13 in]
      }
      frame "Macro: Analiza Pythongowa" {
        # "Initialization Macro\n(This is called once, when the VI starts)"
        n74 = call <vilib>:"Add State(s) to Queue__JKI_lib_State_Machine.vi"("State(s) in Front (\"\")"="Action: Load Image\nAction: Pythong Analyze\nAction: Draw Boundling Box\nAction: SendToDataBase\nUI: Update", "State(s) in (\"\")"=w222) -> ("States Out"=w221:string)  [unwired: 13 in]
      }
      frame "Macro: Analiza zwykla" {
        # "Initialization Macro\n(This is called once, when the VI starts)"
        n75 = call <vilib>:"Add State(s) to Queue__JKI_lib_State_Machine.vi"("State(s) in Front (\"\")"="Action: Load Image\nAction: Analyze Image\nAction: Draw Boundling Box\nAction: SendToDataBase \nUI: Update", "State(s) in (\"\")"=w227) -> ("States Out"=w226:string)  [unwired: 13 in]
      }
      frame "Macro: Exit" {
        # "Exit Macro\n(This is called once, when the VI exits)"
        n76 = Unbundle By Name(w229) -> ("Core.Close Panel on Exit?"=w228:bool)
        n77 = Select(t="UI: Front Panel State >> Close", s=w228, f="") -> (s? t:f=w232:string)
        n78 = call <vilib>:"Add State(s) to Queue__JKI_lib_State_Machine.vi"("State(s) in (\"\")"=w232, "State(s) at Back (\"\")"="Data: Cleanup\nExit") -> ("States Out"=w230:string)  [unwired: 13 in]
        n79 = call <vilib>:"Add State(s) to Queue__JKI_lib_State_Machine.vi"("State(s) in Front (\"\")"=w230, "State(s) in (\"\")"=w237) -> ("States Out"=w236:string)  [unwired: 13 in]
      }
      frame "---------- Action ----------" {
        # "Template Separator\n(You can make a copy of, or modify, this frame)"
        n80 = call <vilib>:"Add State(s) to Queue__JKI_lib_State_Machine.vi"("State(s) in (\"\")"=w241) -> ("States Out"=w240:string)  [unwired: 14 in]
      }
      frame "Action: Pythong Analyze" {
        (unwired) "C:\\\\Users\\\\kacpe\\\\Desktop\\\\OSP\\\\dataset\\\\g6.jpg"
        (unwired) path "C:/Users/kacpe/Documents/LabVIEW Data/ImageProject/scripts/green.py" ("module path")
        n81 = Unbundle By Name(w264) -> ("Input Path"=w263:path)
        n82 = call <vilib>:"Application Directory.vi"() -> ("Application Directory"=w255:path)
        n83 = call <vilib>:"Application Directory.vi"() -> ("Application Directory"=w275:path)
        n84 = Build Path(base path=w255, name or relative path="scripts\\cords.py") -> (appended path=w253:path)
        n85 = Build Path(base path=w275, name or relative path="scripts\\name.py") -> (appended path=w262:path)
        n86 = Path To String(path=w263) -> (string=w250:string)
        n87 = Open Python Session(python version="3.9" ("Python version")) -> (session out=w243:refnum<k35>)  [unwired: 2 in, 1 out]
        n88 = Open Python Session(python version="3.9" ("Python version"), 3:w269) -> (session out=w271:refnum<k35>, error out=w268:errorcluster)  [unwired: 1 in]
        n89 = Build Array(0.0) -> (w251:dbl[])
        n90 = node(w243, w253, "Analyze" ("function name"), w251, w250) -> (w252:refnum<k35>, w249:dbl[])  [unwired: 2 in, 3 out]
        n91 = node(w271, w262, "Analyze" ("function name"), w268, w250, w250) -> (w270:refnum<k35>, w267:errorcluster, w256:string)  [unwired: 1 in, 2 out]
        n92 = Close Python Session(session in=w252) -> ()  [unwired: 1 in, 1 out]
        n93 = Close Python Session(session in=w270, error in=w267) -> (11:w266:errorcluster)
        n94 = Index Array(array=w249, index #1=0 ("index"), index #2=1 ("index"), index #3=2 ("index"), index #4=3 ("index")) -> (element #1=w248:dbl, element #2=w247:dbl, element #3=w246:dbl, element #4=w245:dbl)
        n95 = Bundle By Name(cluster=w264, "Znak"=w256, "Python cords.Left"=w248, "Python cords.Top"=w247, "Python cords.Right"=w246, "Python cords.Bottom"=w245) -> (w265:T9)
      }
      frame "Action: Draw Boundling Box" {
        # "Template Separator\n(You can make a copy of, or modify, this frame)"
        n96 = Unbundle By Name(w283) -> ("Obraz"=w289:T2, "Rectangles"=w281:T10, "Circles"=w280:T7, "Znak"=w282:string, "Matches (pixel)"=w278:T6, "Python cords"=w277:T5)
        n97 = case shown="\"Znak ostrzegawczy\"" w282 {
          tunnel: w281 -> [w293 _ _ _ _]
          tunnel: w280 -> [_ _ _ _ w311]
          tunnel: [w292 T5 {"Left"=0, "Top"=0, "Right"=0, "Bottom"=0} ("output cluster") w295 w300 w310] -> w279
          tunnel: w278 -> [_ _ _ w309 _]
          tunnel: w277 -> [_ _ w295 _ _]
          frame "Znak informacyjny" {
            n98 = call "rectangleBox.vi"("Rectangles 2"=w293) -> ("output cluster"=w292:T5)
          }
          frame "Nie rozpoznano znaku !" {
          }
          frame "", Default {
          }
          frame "Znak ostrzegawczy" {
            n99 = Index Array(array=w309, index #1=0 ("index"), index #2=2 ("index")) -> (element #1=w306:T12, element #2=w305:T12)
            n100 = Unbundle By Name(w305) -> ("Bounding Box"=w304:cluster{"x":sgl, "y":sgl}[])
            n101 = Unbundle By Name(w306) -> ("Position.x"=w299:sgl, "Position.y"=w298:sgl)
            n102 = Index Array(array=w304, index=0) -> (element=w302:cluster{"x":sgl, "y":sgl})
            n103 = Unbundle By Name(w302) -> ("x"=w297:sgl, "y"=w296:sgl)
            n104 = Bundle By Name(cluster=T5 {"Left"=0, "Top"=0, "Right"=0, "Bottom"=0} ("output cluster"), "Left"=w299, "Top"=w298, "Right"=w297, "Bottom"=w296) -> (w300:T5)
          }
          frame "Znak nakazu lub zakazu" {
            n105 = call "circleBox.vi"("Circles 3"=w311) -> ("output cluster"=w310:T5)
          }
        }
        n106 = call "IMAQ Overlay Rectangle"("Color"=u32 16711680, "error in (no error)"=w287, "Rectangle"=w279, "Image"=w289) -> ("error out"=w288:errorcluster, "Image Out"=w285:T2)  [unwired: 6 in]
        n107 = Bundle By Name(cluster=w283, "Obraz"=w285) -> (w284:T9)
        n108 = call <vilib>:"Add State(s) to Queue__JKI_lib_State_Machine.vi"("State(s) in (\"\")"=w291) -> ("States Out"=w290:string)  [unwired: 14 in]
      }
      frame "Action: Analyze Image" {
        w316 = cluster{"Lower value":i32, "Upper value":i32} {"Lower value"=0, "Upper value"=255} ("Red or Hue Range")
        w320 = 2 items=["Red", "Green", "Blue", "Hue", "Saturation", "Luminance", "Value", "Intensity"] ("Color Plane")
        w330 = u16 0 items=["RGB", "HSL", "HSV", "HSI"] ("Color Mode")
        w338 = 0 items=["Red", "Green", "Blue", "Hue", "Saturation", "Luminance", "Value", "Intensity"] ("Color Plane")
        w341 = T13 {"Rotation"=TRUE, "Scale"=TRUE, "Occlusion"=TRUE, "Range Settings"=[]} ("Match Options")
        # "Template Separator\n(You can make a copy of, or modify, this frame)"
        n109 = call <vilib>:"Application Directory.vi"() -> ("Application Directory"=w323:path)
        n110 = Build Path(base path=w323, name or relative path="templates/tringleEx.png") -> (appended path=w321:path)
        n111 = call "IMAQ GetFileInfo"("File Path"=w321) -> ("Image Type"=w347:T15)  [unwired: 4 in, 6 out]
        n112 = call "IMAQ Create"("Image Name"="template", "Image Type"=w347) -> ("New Image"=w346:T2)  [unwired: 3 in, 1 out]
        n113 = call "IMAQ ReadFile 2"("File Path"=w321, "Image"=w346) -> ("Image Out"=w313:T2)  [unwired: 5 in, 4 out]
        n114 = call "IMAQ Create"("Image Name"="blue") -> ("New Image"=w314:T2)  [unwired: 4 in, 1 out]
        n115 = call "IMAQ Copy"("Image Dst"=w314, "Image Src"=w313) -> ("Image Dst Out"=w312:T2)  [unwired: 4 in, 1 out]
        n116 = call "IMAQ ExtractSingleColorPlane"("Color Plane"=w320, "Image Src"=w312) -> ("error out"=w318:errorcluster, "Image Dst Out"=w319:T2)  [unwired: 8 in]
        n117 = call "IMAQ AutoBThreshold 2"("Image Src"=w319, "error in (no error)"=w318) -> ("Threshold Range Out"=w317:cluster{"Lower value":sgl, "Upper value":sgl})  [unwired: 11 in, 2 out]
        n118 = call "IMAQ ColorThreshold"("Blue or Luma or Val or Inten Range"=w317, "Replace Value"=1, "Green or Sat Range"=w316, "Color Mode"=w330, "Red or Hue Range"=w316, "Image Src"=w313) -> ("Image Dst Out"=w328:T2)  [unwired: 4 in, 1 out]
        n119 = call <vilib>:"Add State(s) to Queue__JKI_lib_State_Machine.vi"("State(s) in (\"\")"=w353) -> ("States Out"=w352:string)  [unwired: 14 in]
        n120 = call "IMAQ Create"("Image Name"="analiza") -> ("New Image"=w344:T2)  [unwired: 4 in, 1 out]
        n121 = Unbundle By Name(w332) -> ("Obraz"=w345:T2)
        n122 = call "IMAQ Copy"("Image Dst"=w344, "Image Src"=w345) -> ("Image Dst Out"=w339:T2)  [unwired: 4 in, 1 out]
        n123 = call "IMAQ ExtractSingleColorPlane"("Color Plane"=w338, "Image Src"=w339) -> ("Image Dst Out"=w327:T2)  [unwired: 8 in, 1 out]
        n124 = call "IMAQ Shape Match Tool"("Tolerance"=0.8, "Image Template"=w328, "Image Src"=w327) -> ("Shape Report"=→"Shape Report":T1, "Number of Matches"=w326:i32)  [unwired: 5 in, 2 out]
        "Triangles" <- w326
        n125 = call-poly "IMAQ Detect Shapes"("Match Options"=w341, "Rectangle Descriptor"=T8 {"Min Width"=40.0, "Max Width"=400.0, "Min Height"=40.0, "Max Height"=400.0}, "Image"=w327) -> ("Number of Matches Returned"=w337:i32, "Rectangles"=w335:T10)  [unwired: 6 in, 1 out]
        "Rectangles" <- w337
        n126 = call-poly "IMAQ Detect Shapes"("Minimum match score"=0.01, "error in (no error)"=w350, "Match Options"=w341, "Circle Descriptor"=cluster{"Min Radius":dbl, "Max Radius":dbl} {"Min Radius"=50.0, "Max Radius"=5000.0}, "Image"=w327) -> ("error out"=w351:errorcluster, "Number of Matches Returned"=w336:i32, "Circles"=w334:T7)  [unwired: 4 in]
        "Circles" <- w336
        n127 = call "detectShape.vi"("circle"=w336, "rectangle"=w337, "triangle"=w326) -> ("String"=w325:string)
        n128 = Bundle By Name(cluster=w332, "Rectangles"=w335, "Circles"=w334, "Znak"=w325) -> (w333:T9)
      }
      frame "Action: Load Image" {
        # "Your code here.\n(You can make a copy of, or modify, this frame)"
        n129 = call "IMAQ GetFileInfo"("File Path"="Input Path") -> ("Image Type"=w360:T15)  [unwired: 4 in, 6 out]
        n130 = call "IMAQ Create"("Image Name"="image", "Image Type"=w360) -> ("New Image"=w359:T2)  [unwired: 3 in, 1 out]
        n131 = call "IMAQ ReadFile 2"("File Path"="Input Path", "Image"=w359) -> ("Image Out"=w357:T2)  [unwired: 5 in, 4 out]
        n132 = Bundle By Name(cluster=w355, "Obraz"=w357, "Input Path"="Input Path") -> (w356:T9)
        n133 = call <vilib>:"Add State(s) to Queue__JKI_lib_State_Machine.vi"("State(s) in (\"\")"=w363) -> ("States Out"=w362:string)  [unwired: 14 in]
      }
      frame "Action: Save Image" {
        # "Your code here.\n(You can make a copy of, or modify, this frame)"
        n134 = Unbundle By Name(w365) -> ("Obraz"=w364:T2)
        n135 = call-poly "IMAQ Write File 2"("error in (no error)"=w367, "File Path"="Output Path", "Image"=w364) -> ("error out"=w368:errorcluster)  [unwired: 7 in, 1 out]
        n136 = call <vilib>:"Add State(s) to Queue__JKI_lib_State_Machine.vi"("State(s) in (\"\")"=w370) -> ("States Out"=w369:string)  [unwired: 14 in]
      }
      frame "Action: SendToDataBase" {
        # "Your code here.\n(You can make a copy of, or modify, this frame)"
        n137 = Unbundle By Name(w373) -> ("Input Path"=w372:path)
        n138 = call-poly <vilib>:"DB Tools Open Connection.vi"("error in (no error)"=w374, "connection information"="RecLab") -> ("error out"=w381:errorcluster, "connection reference"=w382:T16)  [unwired: 6 in]
        n139 = Path To String(path=w372) -> (string=w371:string)
        n140 = call <vilib>:"DB Tools Create Parameterized Query.vi"("error in (no error)"=w381, "SQL query"="Parameterized SQL query", "connection reference"=w382) -> ("error out"=w387:errorcluster, "command reference"=w390:T17)  [unwired: 4 in, 1 out]
        n141 = Unbundle By Name(w373) -> ("Znak"=w376:string)
        n142 = call-poly <vilib>:"DB Tools Set Parameter Value.vi"("error in (no error)"=w387, "value"=w371, "parameter index"=0, "command reference"=w390) -> ("error out"=w389:errorcluster, "command reference out"=w388:T17)  [unwired: 4 in]
        n143 = call-poly <vilib>:"DB Tools Set Parameter Value.vi"("error in (no error)"=w389, "value"=w376, "parameter index"=1, "command reference"=w388) -> ("error out"=w377:errorcluster, "command reference out"=w378:T17)  [unwired: 4 in]
        n144 = call-poly <vilib>:"DB Tools Execute Query.vi"("error in (no error)"=w377, "command reference"=w378) -> ("error out"=w391:errorcluster, "command-recordset reference"=w392:T18)  [unwired: 6 in]
        n145 = call-poly <vilib>:"DB Tools Free Object.vi"("error in (no error)"=w391, "command-recordset reference"=w392) -> ("error out"=w385:errorcluster, "command reference"=w393:T17)  [unwired: 8 in]
        n146 = call-poly <vilib>:"DB Tools Free Object.vi"("error in (no error)"=w385, "command reference"=w393) -> ("error out"=w379:errorcluster, "connection reference"=w380:T16)  [unwired: 8 in]
        n147 = call <vilib>:"DB Tools Close Connection.vi"("error in (no error)"=w379, "connection reference"=w380) -> ("error out"=w394:errorcluster)  [unwired: 5 in]
        n148 = call <vilib>:"Simple Error Handler.vi"("error in (no error)"=w394) -> ("error out"=w375:errorcluster)  [unwired: 4 in, 4 out]
        n149 = call <vilib>:"Add State(s) to Queue__JKI_lib_State_Machine.vi"("State(s) in (\"\")"=w397) -> ("States Out"=w396:string)  [unwired: 14 in]
      }
      frame "Action: Clear Image" {
        # "Your code here.\n(You can make a copy of, or modify, this frame)"
        n150 = Bundle By Name(cluster=w400, "Obraz"=T2 refnum, "Znak"="") -> (w401:T9)
        n151 = call <vilib>:"Add State(s) to Queue__JKI_lib_State_Machine.vi"("State(s) in Front (\"\")"="UI: Update" ("State(s) in Front (\"\")"), "State(s) in (\"\")"=w405) -> ("States Out"=w404:string)  [unwired: 13 in]
      }
    }
  }
